vi "Script Get Module Name.vi"(8 "error in":errorcluster, 10 "VI Path":path, 11 "Application in":refnum<vi>) -> (0 "error out":errorcluster, 3 "Module Name":string)   [LabVIEW 2019, in "Panther Dashboard.lvlib"]
uses:
  Panther Dashboard.lvlib
  <vilib>/Utility/traverseref.llb/TRef TravTarget.ctl
  <vilib>/Utility/traverseref.llb/VI Scripting - Traverse.lvlib
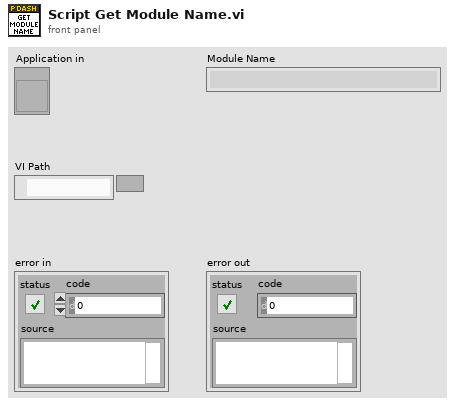
[diagram p1: front panel]
types:
  T1 = typedef "TRef TravTarget.ctl" = enum16{"FP", "BD", "Other"}
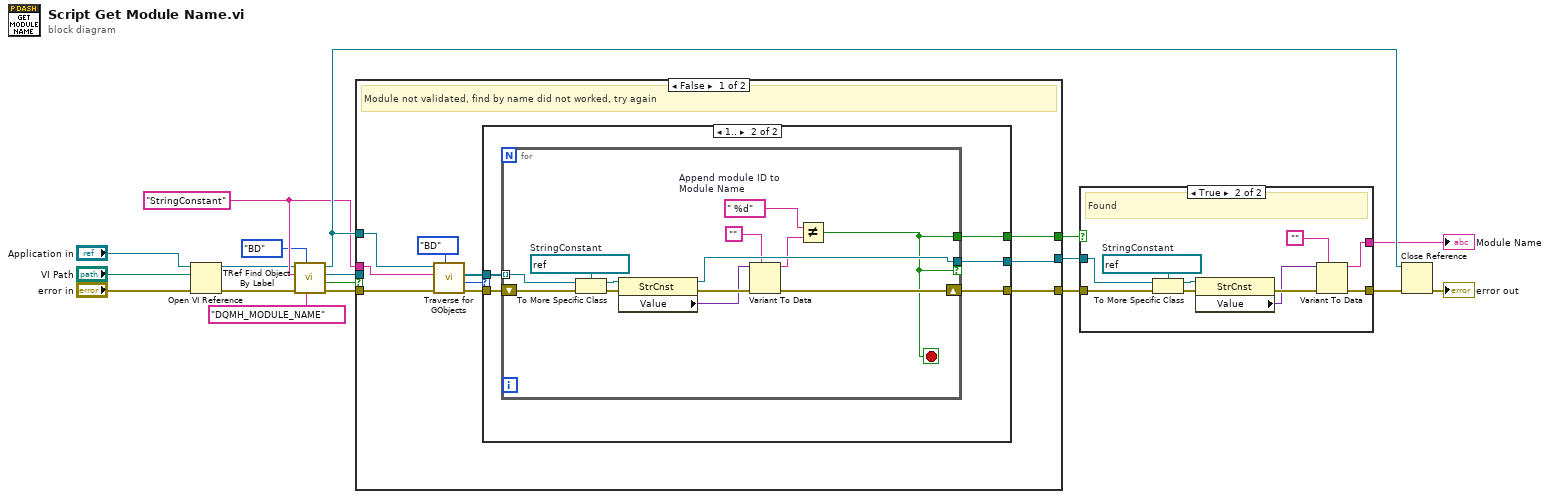
[diagram p0: block diagram]
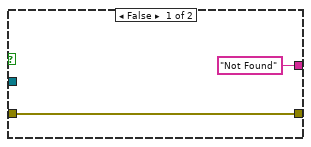
[diagram p2: hidden frame]
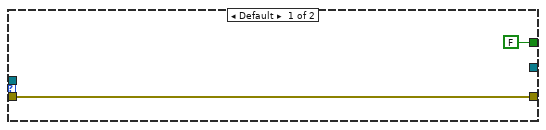
[diagram p3: hidden frame]
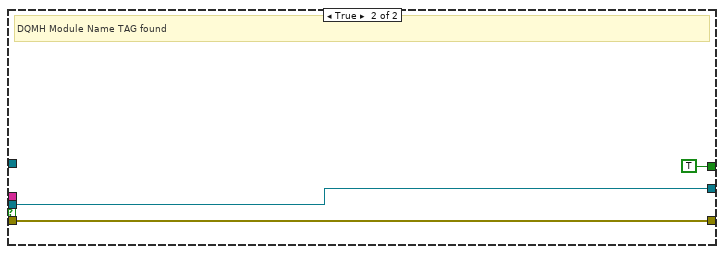
[diagram p4: hidden frame]
diagram:
  w8 = "StringConstant" ("Class Name")
  n1 = Open VI Reference(application reference (local)="Application in", vi path="VI Path", error in (no error)="error in") -> (vi reference=w6:refnum<vi>, error out=w15:errorcluster)  [unwired: 3 in]
  n2 = call <vilib>:"TRef Find Object By Label.vi"("Label"="DQMH_MODULE_NAME", "Traverse Target"=TRef_TravTarget."BD", "error in (no error)"=w15, "Class Name"=w8, "VI Ref"=w6) -> ("error out"=w13:errorcluster, "Found?"=w3:bool, "Found Obj Ref"=w10:refnum<vi>, "dup VI Ref"=w12:refnum<vi>)  [unwired: 3 in]
  n3 = case shown="False" w3 {
    tunnel: w13 -> [w28 w51]
    tunnel: w12 -> [w25 _]
    tunnel: w8 -> [w23 _]
    tunnel: [w26 w51] -> w18
    tunnel: [w19 w50] -> w9
    tunnel: w10 -> [_ w50]
    tunnel: [w20 TRUE] -> w11
    frame False {
      # "Module not validated, find by name did not worked, try again"
      n4 = call <vilib>:"Traverse for GObjects.vi"("Traverse Target"=TRef_TravTarget."BD", "error in (no error)"=w28, "Class Name"=w23, "VI Refnum"=w25) -> ("error out"=w27:errorcluster, "# of Refs"=w22:i32, "References"=w21:refnum<vi>[])  [unwired: 4 in, 1 out]
      n5 = case shown="1.." w22 {
        tunnel: w27 -> [w30 w35]
        tunnel: w21 -> [_ w33]
        tunnel: [w30 w34] -> w26
        tunnel: [FALSE w31] -> w20
        tunnel: [_ w32] -> w19
        frame Default {
        }
        frame 1.. {
          n6 = for {
            tunnel: w33 -> [w42] mode=indexing
            shift-right: [w45] -> w34
            shift-left: w35 -> [w47]
            tunnel: [w41] -> w32 if=w36
            tunnel: [w36] -> w31
            stop <- w36 stop-if-true
            w37 = " %d"  # Append module ID to  Module Name
            w43 = refnum<vi> refnum  # StringConstant
            n7 = To More Specific Class(target class=w43, reference=w42, error in=w47) -> (specific class reference=w44:refnum<vi>, error out=w48:errorcluster)
            n8 = property class="StrCnst"(reference=w44, error in=w48) -> (reference out=w41:refnum<vi>, error out=w46:errorcluster, "Value"=w40:variant)
            n9 = Variant To Data(error in=w46, type="", Variant=w40) -> (data=w38:string, error out=w45:errorcluster)
            n10 = Not Equal?(x=w37, y=w38) -> (x != y?=w36:bool)
          }
        }
      }
    }
    frame True {
      # "DQMH Module Name TAG found"
    }
  }
  n11 = case shown="True" w11 {
    tunnel: [w53 w61] -> w17
    tunnel: ["Not Found" w55] -> w1
    tunnel: w18 -> [w53 w60]
    tunnel: w9 -> [_ w54]
    frame False {
    }
    frame True {
      w56 = refnum<vi> refnum  # StringConstant
      # "Found"
      n12 = To More Specific Class(target class=w56, reference=w54, error in=w60) -> (specific class reference=w58:refnum<vi>, error out=w62:errorcluster)
      n13 = property class="StrCnst"(reference=w58, error in=w62) -> (error out=w63:errorcluster, "Value"=w59:variant)  [unwired: 1 out]
      n14 = Variant To Data(error in=w63, type="", Variant=w59) -> (data=w55:string, error out=w61:errorcluster)
    }
  }
  "Module Name" <- w1
  n15 = Close Reference(reference=w12, error in (no error)=w17) -> (error out=→"error out":errorcluster)
